vi "Train_Artificial Neural Network.vi"(8 "error in (no error)":errorcluster, 10 "UserSettingsESN":T3={"output to internal feedback?"=FALSE, "output to output feedback?"=FALSE, " input to output feedforward?"=TRUE, "number of input (K)"=2, "number of internal (N)"=25, "number of output (L)"=2}, 11 "Data":dbl[][](array[numeric])=array2602x4[10408 elements]) -> (0 "error out":errorcluster, 1 "MSE":dbl, 2 "Wr":dbl[][](graph), 3 "Wl":dbl[][](graph), 5 "ESN trained":T1)   [LabVIEW 2017]
uses:
  ESN network/UserSettingsESN.ctl
  ESN network/ESN_Network.ctl
  <vilib>/Analysis/Matrix/Datatypes/RealMatrix.ctl
  ESN network/ESN_evaluateByMSE(2D array).vi
  <vilib>/Analysis/Matrix/NI_Matrix.lvlib
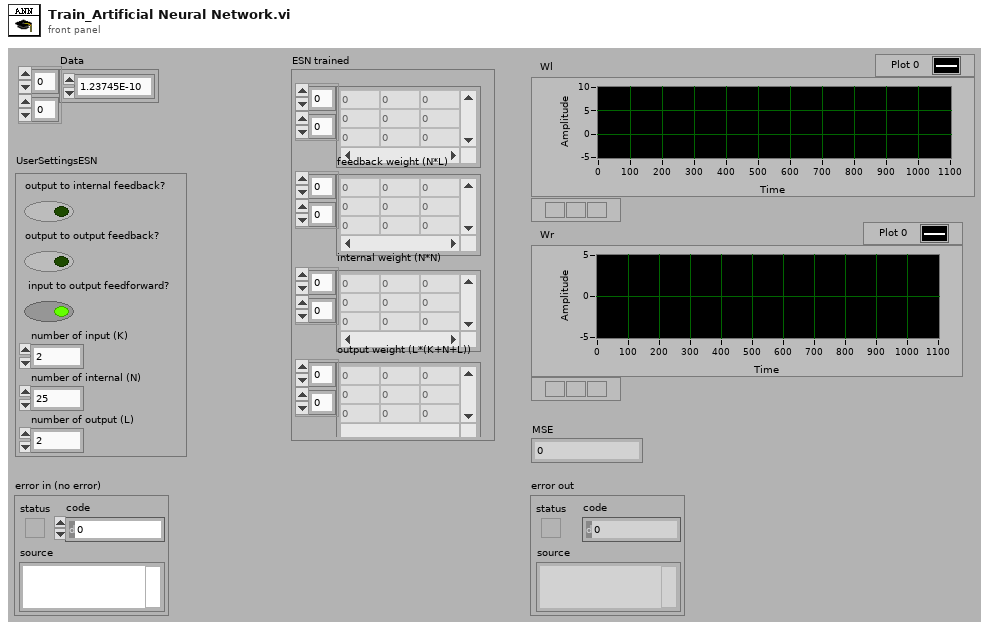
[diagram p1: front panel]
types:
  T1 = typedef "ESN_Network.ctl" = cluster{"output to internal feedback?":bool, "output to output feedback?":bool, "input to output feedforward?":bool, "number of input (K)":i32, "number of internal (N)":i32, "number of output (L)":i32, "input normalization vector":dbl[], "output restore vector":dbl[], "input weight (N*K)":T2, "feedback weight (N*L)":T2, "internal weight (N*N)":T2, "output weight (L*(K+N+L))":T2}
  T2 = typedef "NI_Matrix.lvlib/RealMatrix.ctl" = dbl[][]
  T3 = typedef "UserSettingsESN.ctl" = cluster{"output to internal feedback?":bool, "output to output feedback?":bool, " input to output feedforward?":bool, "number of input (K)":i32, "number of internal (N)":i32, "number of output (L)":i32}
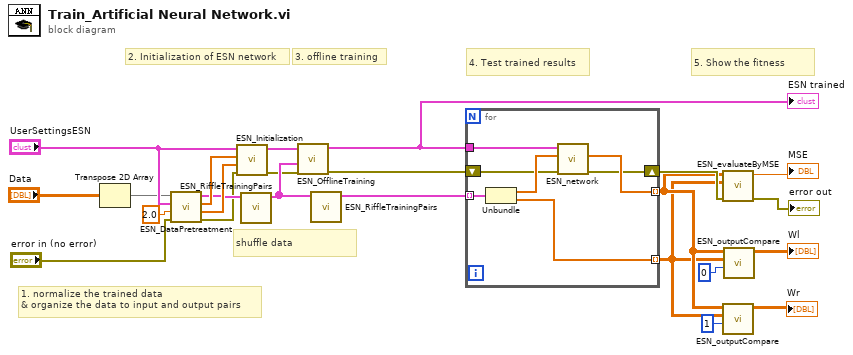
[diagram p0: block diagram]
diagram:
  # "5. Show the fitness"
  # "4. Test trained results"
  # "shuffle data"
  # "3. offline training"
  # "2. Initialization of ESN network"
  # "1. normalize the trained data\n& organize the data to input and output pairs"
  n1 = Transpose 2D Array(2D array="Data") -> (transposed array=w17:dbl[][])
  n2 = call "ESN_DataPretreatment.vi"("error in (no error)"="error in (no error)", "Scale factor (2)"=2.0, "UserSettingsESN"="UserSettingsESN", "Data"=w17) -> ("error out"=w8:errorcluster, "output restore vector"=w22:dbl[], "input normalization vector"=w23:dbl[], "I/O pairs"=w15:cluster{dbl[], dbl[]}[])  [unwired: 4 in]
  n3 = call "ESN_Initialization.vi"("error in (no error)"=w8, "output normalization vector"=w22, "input normalization vector"=w23, "UserSettingsESN"="UserSettingsESN") -> ("error out"=w11:errorcluster, "ESN Status"=w12:T1)  [unwired: 6 in]
  n4 = call "ESN_RiffleTrainingPairs.vi"("Input output pairs"=w15) -> ("Input output pairs"=w16:cluster{"Input":dbl[], "Output":dbl[]}[])  [unwired: 10 in]
  n5 = call "ESN_OfflineTraining.vi"("error in (no error)"=w11, "I/O pairs"=w16, "ESN Status"=w12) -> ("error out"=w7:errorcluster, "ESN trained"=w14:T1)  [unwired: 7 in]
  "ESN trained" <- w14
  n6 = call "ESN_RiffleTrainingPairs.vi"("Input output pairs"=w16) -> ("Input output pairs"=w13:cluster{"Input":dbl[], "Output":dbl[]}[])  [unwired: 10 in]
  n7 = for {
    tunnel: w14 -> [w31]
    tunnel: w13 -> [w30] mode=indexing
    tunnel: [w28] -> w4 mode=indexing
    tunnel: [w27] -> w3 mode=indexing
    shift-right: [w25] -> w6
    shift-left: w7 -> [w26]
    n8 = Unbundle(w30) -> ("Input"=w29:dbl[], "Output"=w27:dbl[])
    n9 = call "ESN_network.vi"("error in (no error)"=w26, "input"=w29, "ESN Status"=w31) -> ("error out"=w25:errorcluster, "output"=w28:dbl[])  [unwired: 5 in, 2 out]
  }
  n10 = call-poly "ESN_evaluateByMSE.vi"("error in (no error)"=w6, "desired Output"=w3, "Output"=w4) -> ("error out"=→"error out":errorcluster, "MSE"=→"MSE":dbl)  [unwired: 7 in]
  n11 = call "ESN_outputCompare.vi"("index (row)"=1, "disired output"=w3, "output"=w4) -> ("Waveform Graph"=→"Wr":dbl[][])  [unwired: 8 in]
  n12 = call "ESN_outputCompare.vi"("index (row)"=0, "disired output"=w3, "output"=w4) -> ("Waveform Graph"=→"Wl":dbl[][])  [unwired: 8 in]
